vi "Initialize.vi"(8 "error in (no error)":errorcluster, 9 "connectionWaitTime(ms)":u32=1000, 10 "Address":u8, 11 "VISA resource name":refnum<visa-resource-name>) -> (0 "error out":errorcluster, 1 "Raw Response":string, 3 "VISA resource name out":refnum<visa-resource-name>)   [LabVIEW 2020, in "driver_flodx_rtd.lvlib"]
doc: "Initializes communication with the device, by opening up a Visa port, and configuring the serial settings."
uses:
  <instrlib>/RxnRover/FloDx RTD Driver/driver_flodx_rtd.lvlib
  <vilib>/Instr/_visa.llb/VISA Open Access Mode.ctl
  <instrlib>/RxnRover/FloDx RTD Driver/Public/Type Defs/SerialConfig.ctl
  <vilib>/Instr/_visa.llb/VISA Configure Serial Port (Instr).vi
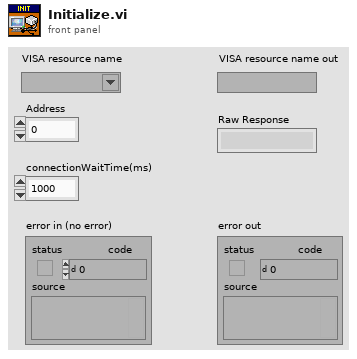
[diagram p1: front panel]
types:
  T1 = typedef "driver_flodx_rtd.lvlib/SerialConfig.ctl" = cluster{"baud rate":u32, "data bits":u16, "parity (0:none)":enum16{"None", "Odd", "Even", "Mark", "Space"}, "Enable Termination\nChar (T/F)":bool, "termination char\n(0xA = '\\n' = LF) ":u8, "stop bits (10: 1 bit)":u16, "flow control (0:none)":u16, "timeout ms":u32}
  T2 = typedef "VISA Open Access Mode.ctl" = u32
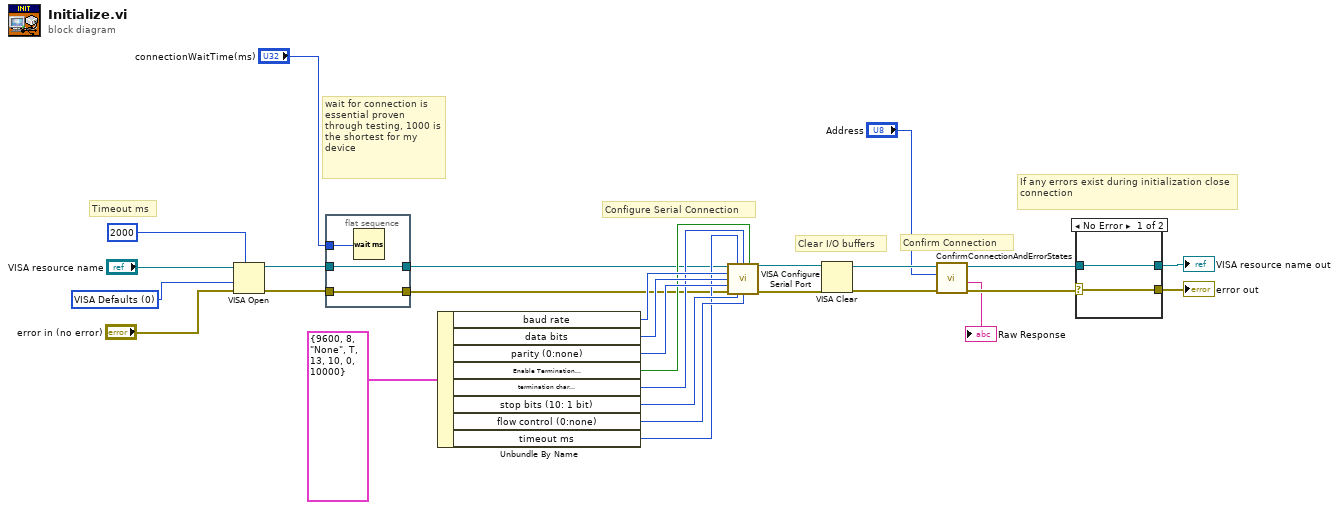
[diagram p0: block diagram]
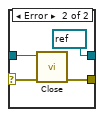
[diagram p2: hidden frame]
diagram:
  w26 = T2 0 items=["VISA Defaults"=0, "Exclusive Lock"=1, "Load Configured Settings"=4] ("Access Mode")
  # "wait for connection is essential proven through testing, 1000 is the shortest for my device"
  # "Confirm Connection"
  # "If any errors exist during initialization close connection"
  # "Configure Serial Connection"
  # "Clear I/O buffers"
  # "Timeout ms"
  n1 = VISA Open(timeout (0)=u32 2000 ("VISA Open timeout (0)"), access mode=w26, error in (no error)="error in (no error)", VISA resource name="VISA resource name") -> (VISA resource name=w6:refnum<visa-resource-name>, error out=w3:errorcluster)  [unwired: 1 in]
  n2 = flat-sequence {
    tunnel: "connectionWaitTime(ms)" -> [w31]
    tunnel: w6 -> [w30]
    tunnel: [w30] -> w5
    tunnel: [w29] -> w4
    tunnel: w3 -> [w29]
    frame #0 {
      n3 = Wait (ms)(milliseconds to wait=w31) -> ()  [unwired: 1 out]
    }
  }
  n4 = Unbundle By Name(T1 {"baud rate"=9600, "data bits"=8, "parity (0:none)"=enum."None", "Enable Termination\nChar (T/F)"=TRUE, "termination char\n(0xA = '\\n' = LF) "=13, "stop bits (10: 1 bit)"=10, "flow control (0:none)"=0, "timeout ms"=10000} ("Serial Configuration")) -> ("baud rate"=w25:u32, "data bits"=w24:u16, "parity (0:none)"=w23:enum16{"None", "Odd", "Even", "Mark", "Space"}, "Enable Termination\nChar (T/F)"=w22:bool, "termination char\n(0xA = '\\n' = LF)"=w21:u8, "stop bits (10: 1 bit)"=w20:u16, "flow control (0:none)"=w19:u16, "timeout ms"=w18:u32)
  n5 = call-poly "VISA Configure Serial Port"("VISA resource name"=w5, "timeout (10sec)"=w18, "termination char\n(0xA = '\\n' = LF)"=w21, "Enable Termination\nChar (T)"=w22, "baud rate (9600)"=w25, "data bits (8)"=w24, "parity (0:none)"=w23, "error in (no error)"=w4, "stop bits (10: 1 bit)"=w20, "flow control (0:none)"=w19) -> ("VISA resource name out"=w17:refnum<visa-resource-name>, "error out"=w16:errorcluster)  [unwired: 4 in]
  n6 = VISA Clear(VISA resource name=w17, error in (no error)=w16) -> (VISA resource name out=w12:refnum<visa-resource-name>, error out=w11:errorcluster)
  n7 = call <instrlib>:"ConfirmConnectionAndErrorStates.vi"("error in (no error)"=w11, "Address"="Address", "VISA resource name"=w12) -> ("error out"=w9:errorcluster, "Raw Response"=→"Raw Response":string, "VISA resource name out"=w8:refnum<visa-resource-name>)  [unwired: 5 in, 1 out]
  n8 = case shown="No Error" w9 {
    selector: w9 -> [w32 w36]
    tunnel: w8 -> [w33 w34]
    tunnel: [w33 refnum<visa-resource-name> refnum ("VISA resource name out")] -> w14
    tunnel: [w32 w35] -> w13
    frame No Error {
    }
    frame Error {
      n9 = call <instrlib>:"Close.vi"("error in (no error)"=w36, "VISA resource name"=w34) -> ("error out"=w35:errorcluster)  [unwired: 9 in]
    }
  }
  "VISA resource name out" <- w14
  "error out" <- w13
